vi "Wolna_generuj_analog_wektory.vi"(8 "error in (no error)":errorcluster, 9 "Przetworzone in":T2, 10 "Wolna In":T3={"WolnaStart"=FALSE, "WolnaPrzeglad"=FALSE, "Okres"=0.02, "Czas max"=120.0, "WolnaKonfiguracja"=FALSE, "Rej.1"={"Typ rejestracji"=enum."Wprost (średnia)", "Kanały"=[1], "Opis"="Rej.X", "Aktywny"=FALSE, "Wolna Wykr num"=0}, "Rej.2"={"Typ rejestracji"=enum."Wprost (średnia)", "Kanały"=[1], "Opis"="Rej.X", "Aktywny"=FALSE, "Wolna Wykr num"=0}, "Rej.3"={"Typ rejestracji"=enum."Wprost (średnia)", "Kanały"=[1], "Opis"="Rej.X", "Aktywny"=FALSE, "Wolna Wykr num"=0}, "Rej.4"={"Typ rejestracji"=enum."Wprost (średnia)", "Kanały"=[1], "Opis"="Rej.X", "Aktywny"=FALSE, "Wolna Wykr num"=0}, "Rej.5"={"Typ rejestracji"=enum."Wprost (średnia)", "Kanały"=[1], "Opis"="Rej.X", "Aktywny"=FALSE, "Wolna Wykr num"=0}, "Rej.6"={"Typ rejestracji"=enum."Wprost (średnia)", "Kanały"=[1], "Opis"="Rej.X", "Aktywny"=FALSE, "Wolna Wykr num"=0}, "Rej.7"={"Typ rejestracji"=enum."Wprost (średnia)", "Kanały"=[1], "Opis"="Rej.X", "Aktywny"=FALSE, "Wolna Wykr num"=0}, "Rej.8"={"Typ rejestracji"=enum."Wprost (średnia)", "Kanały"=[1], "Opis"="Rej.X", "Aktywny"=FALSE, "Wolna Wykr num"=0}} {"Rej.8"."Wolna Wykr num" items=["Brak", "Wykres 1", "Wykres 2", "Wykres 3", "Wykres 4"]; "Rej.7"."Wolna Wykr num" items=["Brak", "Wykres 1", "Wykres 2", "Wykres 3", "Wykres 4"]; "Rej.6"."Wolna Wykr num" items=["Brak", "Wykres 1", "Wykres 2", "Wykres 3", "Wykres 4"]; "Rej.5"."Wolna Wykr num" items=["Brak", "Wykres 1", "Wykres 2", "Wykres 3", "Wykres 4"]; "Rej.4"."Wolna Wykr num" items=["Brak", "Wykres 1", "Wykres 2", "Wykres 3", "Wykres 4"]; "Rej.3"."Wolna Wykr num" items=["Brak", "Wykres 1", "Wykres 2", "Wykres 3", "Wykres 4"]; "Rej.2"."Wolna Wykr num" items=["Brak", "Wykres 1", "Wykres 2", "Wykres 3", "Wykres 4"]; "Rej.1"."Wolna Wykr num" items=["Brak", "Wykres 1", "Wykres 2", "Wykres 3", "Wykres 4"]; "Czas max" min=2.0; "Okres" min=0.001}, 11 "Restart In":bool) -> (0 "error out":errorcluster, 1 "Przetworzone out":T2, 2 "Rej Param":cluster{"Kanały":i32[][], T1[]})   [LabVIEW 2014]
doc: "Przy restarcie akwizycji wolnej\nGeneruje wektory akwizychi\nna podstawie liczby kanałów rejestrowanych"
uses:
  Kontrolki/GUI/Rejestracja_wolna.ctl
  Kontrolki/GUI/RejWol_konfig.ctl
  Kontrolki/GUI/RejWol_typ.ctl
  Kontrolki/GUI/Wolna_WykrNum.ctl
  Kontrolki/Przetwarzanie/Kanaly.ctl
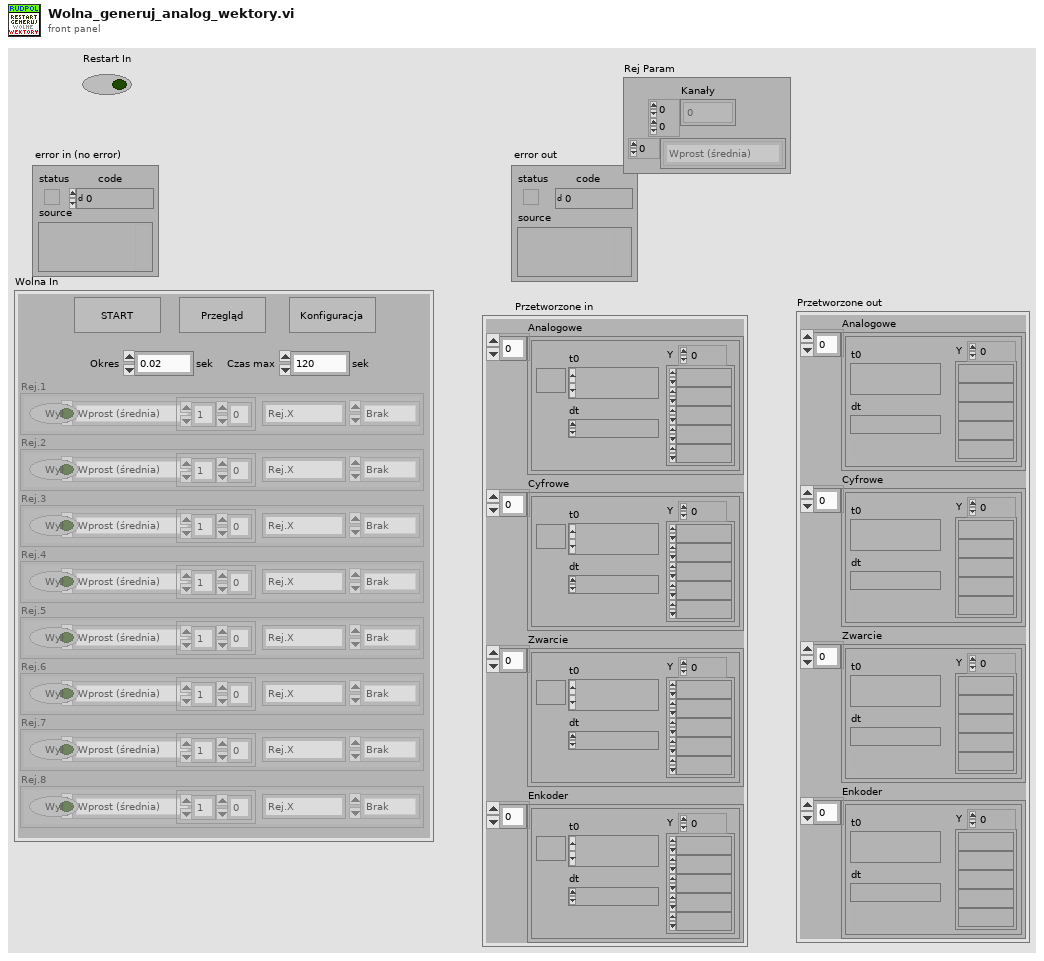
[diagram p1: front panel]
types:
  T1 = typedef "RejWol_typ.ctl" = enum16{"Wprost (średnia)", "Moduł (śr. wypr)", "Kwadrat (skuteczna)", "Iloczyn", "Faza"}
  T2 = typedef "Kanaly.ctl" = cluster{"Analogowe":waveform(dbl)[], "Cyfrowe":waveform(dbl)[], "Zwarcie":waveform(dbl)[], "Enkoder":waveform(dbl)[]}
  T3 = typedef "Rejestracja_wolna.ctl" = cluster{"WolnaStart":bool, "WolnaPrzeglad":bool, "Okres":dbl, "Czas max":dbl, "WolnaKonfiguracja":bool, "Rej.1":T4, "Rej.2":T4, "Rej.3":T4, "Rej.4":T4, "Rej.5":T4, "Rej.6":T4, "Rej.7":T4, "Rej.8":T4}
  T4 = typedef "RejWol_konfig.ctl" = cluster{"Typ rejestracji":T1, "Kanały":i32[], "Opis":string, "Aktywny":bool, "Wolna Wykr num":T5}
  T5 = typedef "Wolna_WykrNum.ctl" = u16
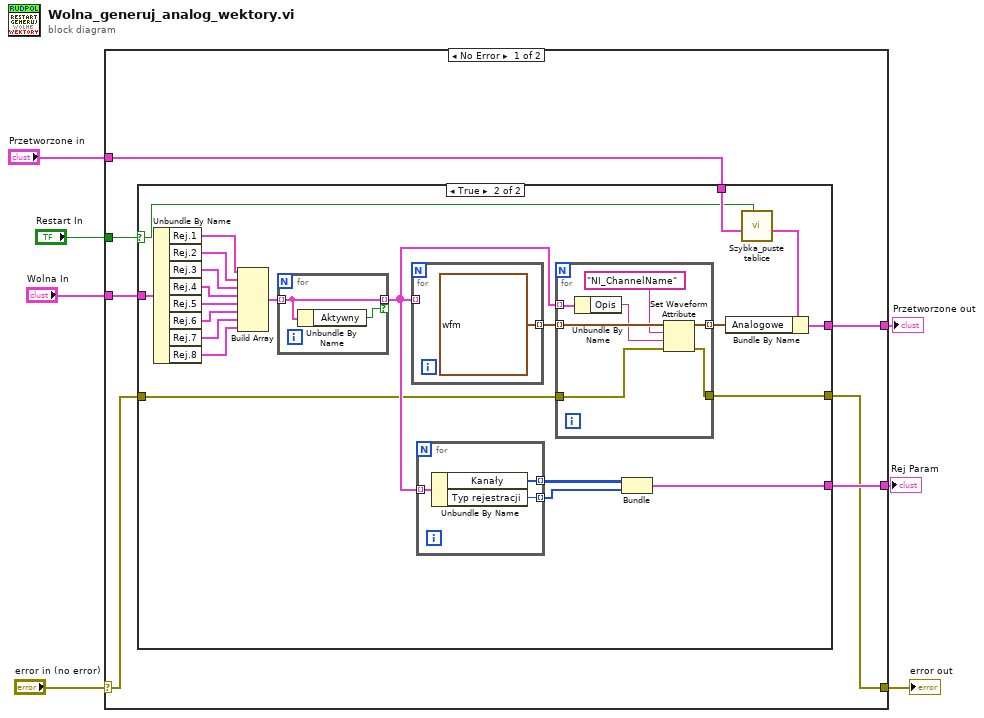
[diagram p0: block diagram]
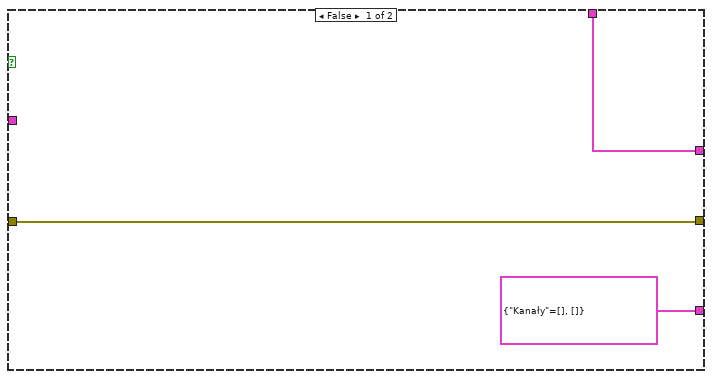
[diagram p2: hidden frame]
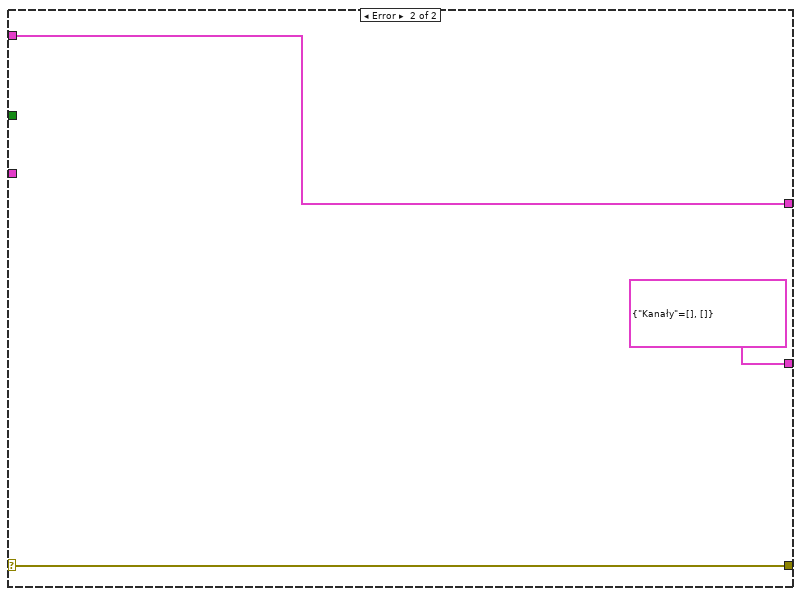
[diagram p3: hidden frame]
diagram:
  n1 = case shown="No Error" "error in (no error)" {
    selector: "error in (no error)" -> [w10 w55]
    tunnel: [w9 w55] -> w6
    tunnel: "Wolna In" -> [w14 _]
    tunnel: "Restart In" -> [w12 _]
    tunnel: [w13 w54] -> w3
    tunnel: "Przetworzone in" -> [w8 w54]
    tunnel: [w11 cluster{"Kanały":i32[][], T1[]} {"Kanały"=[], []}] -> w1
    frame No Error {
      n2 = case shown="True" w12 {
        selector: w12 -> [_ w18]
        tunnel: w14 -> [_ w39]
        tunnel: [w15 w29] -> w13
        tunnel: [cluster{"Kanały":i32[][], T1[]} {"Kanały"=[], []} w26] -> w11
        tunnel: w10 -> [w16 w22]
        tunnel: [w16 w21] -> w9
        tunnel: w8 -> [w15 w19]
        frame False {
        }
        frame True {
          n3 = Unbundle By Name(w39) -> ("Rej.1"=w38:T4, "Rej.2"=w37:T4, "Rej.3"=w36:T4, "Rej.4"=w35:T4, "Rej.5"=w34:T4, "Rej.6"=w33:T4, "Rej.7"=w32:T4, "Rej.8"=w31:T4)
          n4 = Build Array(w38, w37, w36, w35, w34, w33, w32, w31) -> (w30:T4[])
          n5 = for {
            tunnel: w30 -> [w52] mode=indexing
            tunnel: [w52] -> w23 mode=indexing if=w51
            n6 = Unbundle By Name(w52) -> ("Aktywny"=w51:bool)
          }
          n7 = for {
            tunnel: [waveform(dbl) {"t0"=timestamp(0 s since 1904-01-01), "dt"=1.0, "Y"=[]} ("Waveform")] -> w25 mode=indexing
            tunnel: w23 -> [_] mode=indexing
          }
          n8 = for {
            tunnel: w23 -> [w49] mode=indexing
            tunnel: [w48] -> w28 mode=indexing
            tunnel: [w47] -> w27 mode=indexing
            n9 = Unbundle By Name(w49) -> ("Kanały"=w48:i32[], "Typ rejestracji"=w47:T1)
          }
          n10 = for {
            tunnel: w25 -> [w46] mode=indexing
            tunnel: [w45] -> w24 mode=indexing
            tunnel: w23 -> [w44] mode=indexing
            tunnel: w22 -> [w41]
            tunnel: [w40] -> w21
            n11 = Unbundle By Name(w44) -> ("Opis"=w43:string)
            n12 = Set Waveform Attribute(4:w41, 5:w43, 6:"NI_ChannelName", 7:w46) -> (0:w40:errorcluster, 3:w45:waveform(dbl))  [unwired: 1 out]
          }
          n13 = Bundle("Kanały"=w28, w27) -> (w26:cluster{"Kanały":i32[][], T1[]})  [unwired: 1 in]
          n14 = call "Szybka_puste tablice.vi"("Reset"=w18, "Bufor in"=w19) -> ("Kanaly out"=w20:T2)  [unwired: 8 in, 1 out]
          n15 = Bundle By Name(cluster=w20, "Analogowe"=w24) -> (w29:T2)
        }
      }
    }
    frame Error {
    }
  }
  "error out" <- w6
  "Przetworzone out" <- w3
  "Rej Param" <- w1
